vi "AnyBuilderBuildToBuffer.vi"(8 "error in":errorcluster, 10 "Message Type":string, 11 "Builder Ref":T1) -> (0 "error out":errorcluster, 3 "Buffer":u8[](array[numeric]))   [LabVIEW 2019, in "grpc-lvsupport.lvlib"]
uses:
  grpc-lvsupport.lvlib
  Shared/grpcId.ctl
  <vilib>/AdvancedString/1D String Array to Delimited String.vi
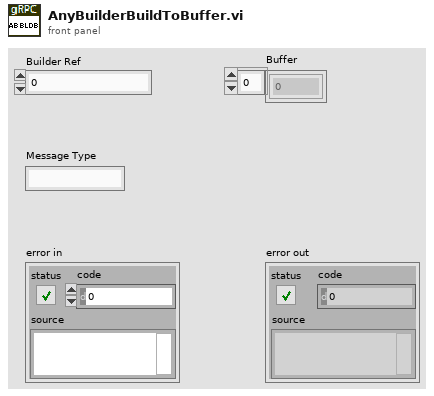
[diagram p1: front panel]
types:
  T1 = typedef "grpc-lvsupport.lvlib/grpcId.ctl" = u64
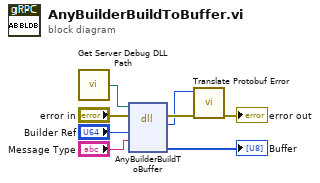
[diagram p0: block diagram]
diagram:
  n1 = call "Get Server Debug DLL Path.vi"() -> ("Server Debug DLL Path"=w6:path)
  n2 = dll-call lib="?" fn="AnyBuilderBuildToBuffer"(path in=w6, error in="error in", "builderId"="Builder Ref", "messageType"="Message Type") -> (error out=w7:errorcluster, "return type"=w1:i32, "anyId"=→"Buffer":u8[])  [unwired: 4 in, 1 out]
  n3 = call "Translate Protobuf Error.vi"("error in"=w7, "Error Code"=w1) -> ("error out"=→"error out":errorcluster)  [unwired: 9 in]
